vi "Launch SessionCore (Server).vi"(8 "error in (no error)":errorcluster, 11 "Session in":refnum<class "Session.lvclass">) -> (0 "error out":errorcluster, 2 "Session ID":i32, 3 "Session out":refnum<class "Session.lvclass">)   [LabVIEW 2013, in "MQTT Server.lvlib" / "Session.lvclass"]
uses:
  Session.lvclass
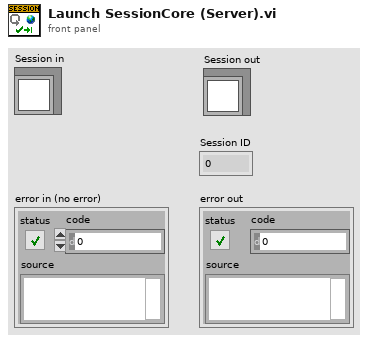
[diagram p1: front panel]
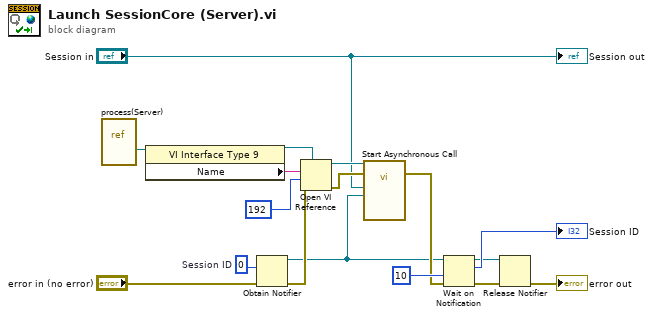
[diagram p0: block diagram]
diagram:
  w8 = 0  # Session ID
  n1 = vi-ref "process(Server).vi"() -> (w2:refnum<vi>)
  n2 = property class="VI Interface Type 9"(reference=w2) -> (reference out=w4:refnum<vi>, "Name"=w3:string)  [unwired: 1 in, 1 out]
  n3 = Obtain Notifier(notification data type=w8, error in (no error)="error in (no error)") -> (notifier out=w9:refnum<notifier>, error out=w14:errorcluster)  [unwired: 2 in, 1 out]
  n4 = Open VI Reference(type specifier VI Refnum (for type only)=w4, vi path=w3, options=192, error in (no error)=w14) -> (vi reference=w5:refnum<vi>, error out=w6:errorcluster)  [unwired: 2 in]
  n5 = call-by-ref "Start Asynchronous Call"(reference=w5, error in=w6, "Sync"=w9, "Session in"="Session in") -> (error out=w12:errorcluster)  [unwired: 8 in, 3 out]
  n6 = Wait on Notification(notifier=w9, timeout in ms (-1)=10, error in (no error)=w12) -> (notifier out=w10:refnum<notifier>, notification=→"Session ID":i32, error out=w13:errorcluster)  [unwired: 1 in, 1 out]
  n7 = Release Notifier(notifier=w10, error in (no error)=w13) -> (error out=→"error out":errorcluster)  [unwired: 1 in, 2 out]
  "Session out" <- "Session in"
